vi "FGVSignalAcquisition.vi"(7 "Enum":T1, 8 "error in":errorcluster, 9 "DataIn":waveform(i16), 10 "ReadIn":bool) -> (0 "error out":errorcluster, 1 "DataOut":waveform(i16), 2 "ReadOut":bool)   [LabVIEW 2016]
uses:
  controls/Enum.ctl
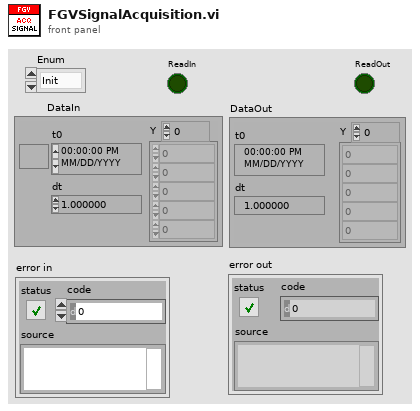
[diagram p1: front panel]
types:
  T1 = typedef "Enum.ctl" = enum16{"Init", "Read", "Write"}
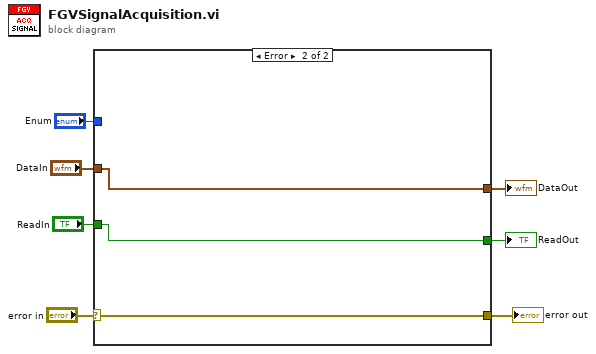
[diagram p0: block diagram]
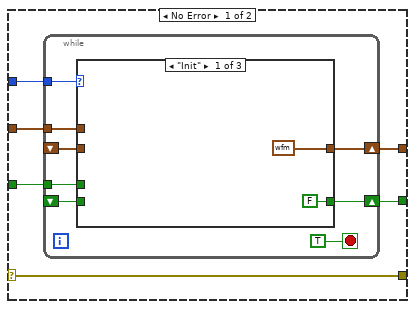
[diagram p2: hidden frame]
diagram:
  n1 = case shown="Error" "error in" {
    selector: "error in" -> [w12 w30]
    tunnel: "Enum" -> [w13 _]
    tunnel: [w12 w30] -> w6
    tunnel: "DataIn" -> [w11 w29]
    tunnel: [w10 w29] -> w4
    tunnel: "ReadIn" -> [w9 w28]
    tunnel: [w8 w28] -> w1
    frame No Error {
      n2 = while {
        tunnel: w13 -> [w20]
        tunnel: w11 -> [w19]
        shift-right: [w18] -> w10
        shift-left: _ -> [w17]
        tunnel: w9 -> [w16]
        shift-right: [w15] -> w8
        shift-left: _ -> [w14]
        stop <- TRUE stop-if-true
        n3 = case shown="\"Init\"" w20 {
          tunnel: w19 -> [_ _ w27]
          tunnel: [waveform(i16) {"t0"=timestamp(0 s since 1904-01-01), "dt"=1.0, "Y"=[]} ("DataIn") w25 w27] -> w18
          tunnel: w17 -> [_ w25 _]
          tunnel: w16 -> [_ _ w26]
          tunnel: [FALSE ("ReadIn") w24 w26] -> w15
          tunnel: w14 -> [_ w24 _]
          frame "Init" {
          }
          frame "Read", Default {
          }
          frame "Write" {
          }
        }
      }
    }
    frame Error {
    }
  }
  "error out" <- w6
  "DataOut" <- w4
  "ReadOut" <- w1
